vi "Main_Measurement.vi"(5 "error in":errorcluster) -> (19 "error out":errorcluster)   [LabVIEW 2011]
uses:
  Camera/lib/atmcd32d.llb/Shutter_type typedef.ctl
  Camera/lib/atmcd32d.llb/Shutter_mode typedef.ctl
  Camera/lib/atmcd32d.llb/Spool_method typedef.ctl
  Camera/lib/atmcd32d.llb/OutputAmplifier_type typedef.ctl
  Camera/lib/atmcd32d.llb/EMGainMode_mode typedef.ctl
  Camera/lib/atmcd32d.llb/Error Code Enum typedef.ctl
  Camera/lib/atmcd32d.llb/AcquisitionMode_mode typedef.ctl
  Camera/lib/atmcd32d.llb/ReadMode_mode typedef.ctl
  Camera/lib/atmcd32d.llb/TriggerMode_mode typedef.ctl
  Utilities/controls/ctlSeqFNs_PI_SysNr.ctl
  Variables/GlobalSetGetPixelOfRoi.vi
  Variables/ScanDirection.vi
  Variables/IlluminationPatterns.vi
  Variables/GlobalSetGetTriggerForPointMeasurement.vi
  Variables/GlobalDevice.vi
  Kinetics/vi/RampOrLin.vi
  Variables/MesaurementType.vi
  Variables/GlobalSetNumberOfDigits_PhysikalInstruments.vi
  Variables/GlobalSetNumberOfDigits_Scanners.vi
  Variables/ccdChipPixels.vi
  Variables/GlobalSetGetConfigureCamera.vi
  Variables/GlobalGetTimingsFromCamera.vi
  Variables/SavPath.vi
  Variables/GlobalSetConfigurationPhysikalInstruments.vi
  Variables/GlobalSetGetPositionParameters.vi
  <vilib>/DAQmx/create/channels.llb/DAQmx Create Channel (CO-Pulse Generation-Frequency).vi
  <vilib>/DAQmx/configure/timing.llb/DAQmx Timing (Implicit).vi
  <vilib>/DAQmx/configure/trigger.llb/DAQmx Start Trigger (Digital Edge).vi
  Variables/Pulsecounter.vi
  Variables/ModulationNiveaus.vi
  Variables/AOTF_NonLinearLinesOnOff.vi
  Variables/MesaurementTime.vi
  Program Files/National Instruments/LabVIEW 2011/resource/objmgr/daqmx.rc
panel:
  out "first":u32
  out "last":i32
  out "ypixels":i32
  out "xpixels":i32
  out "keepCleanTime":sgl
types:
  T1 = enum32{"Non Linear Illumniation", "Constant Illumination"}
  T2 = typedef "Shutter_type typedef.ctl" = enum16{"TTL Low", "TTL High"}
  T3 = typedef "Shutter_mode typedef.ctl" = enum16{"Auto", "Open", "Close"}
  T4 = typedef "Spool_method typedef.ctl" = enum16{"32-bit", "Depends", "16-bit", "Multiple Directory", "Spool to RAM disk", "16-bit FITS", "SIF", "16-buit TIFF", "Multiple Directory Compressed"}
  T5 = typedef "Error Code Enum typedef.ctl" = enum32{"N/A (0)", "DRV_ERROR_CODES", "DRV_SUCCESS", "DRV_VXDNOTINSTALLED", "DRV_ERROR_SCAN", "DRV_ERROR_CHECK_SUM", "DRV_ERROR_FILELOAD", "DRV_UNKNOWN_FUNC", "DRV_ERROR_VXD_INIT", "DRV_ERROR_ADDRESS", "DRV_ERROR_PAGELOCK", "DRV_ERROR_PAGEUNLOCK", "DRV_ERROR_BOARDTEST", "DRV_ERROR_ACK", "DRV_ERROR_UP_FIFO", "DRV_ERROR_PATTERN", "N/A (16)", "DRV_ACQUISITION_ERRORS", "DRV_ACQ_BUFFER", "DRV_ACQ_DOWNFIFO_FULL", "DRV_PROC_UNKONWN_INSTRUCTION", "DRV_ILLEGAL_OP_CODE", "DRV_KINETIC_TIME_NOT_MET", "DRV_ACCUM_TIME_NOT_MET", "DRV_NO_NEW_DATA", "N/A (25)", "DRV_SPOOLERROR", "N/A (27)", "N/A (28)", "N/A (29)", "N/A (30)", "N/A (31)", "N/A (32)", "DRV_TEMPERATURE_CODES", "DRV_TEMPERATURE_OFF", "DRV_TEMPERATURE_NOT_STABILIZED", "DRV_TEMPERATURE_STABILIZED", "DRV_TEMPERATURE_NOT_REACHED", "DRV_TEMPERATURE_OUT_RANGE", "DRV_TEMPERATURE_NOT_SUPPORTED", "DRV_TEMPERATURE_DRIFT", "N/A (41)", "N/A (42)", "N/A (43)", "N/A (44)", "N/A (45)", "N/A (46)", "N/A (47)", "N/A (48)", "DRV_GENERAL_ERRORS", "DRV_INVALID_AUX", "DRV_COF_NOTLOADED", "DRV_FPGAPROG", "DRV_FLEXERROR", "DRV_GPIBERROR", "N/A (55)", "N/A (56)", "N/A (57)", "N/A (58)", "N/A (59)", "N/A (60)", "N/A (61)", "N/A (62)", "N/A (63)", "DRV_DATATYPE", "DRV_DRIVER_ERRORS", "DRV_P1INVALID", "DRV_P2INVALID", "DRV_P3INVALID", "DRV_P4INVALID", "DRV_INIERROR", "DRV_COFERROR", "DRV_ACQUIRING", "DRV_IDLE", "DRV_TEMPCYCLE", "DRV_NOT_INITIALIZED", "DRV_P5INVALID", "DRV_P6INVALID", "DRV_INVALID_MODE", "DRV_INVALID_FILTER", "DRV_I2CERRORS", "DRV_I2CDEVNOTFOUND", "DRV_I2CTIMEOUT", "DRV_P7INVALID", "N/A (84)", "N/A (85)", "N/A (86)", "N/A (87)", "N/A (88)", "N/A (89)", "DRV_IOCERROR", "DRV_VRMVERSIONERROR"}
  T6 = typedef "OutputAmplifier_type typedef.ctl" = enum16{"Standard EMCCD gain register", "Conventional CCD register"}
  T7 = typedef "EMGainMode_mode typedef.ctl" = enum16{"8-bit", "12-bit", "Linear", "Real"}
  T8 = typedef "TriggerMode_mode typedef.ctl" = enum16{"Internal", "External", "N/A (2)", "N/A (3)", "N/A (4)", "N/A (5)", "External Start"}
  T9 = typedef "AcquisitionMode_mode typedef.ctl" = enum16{"Reserved (0)", "Single Scan", "Accumulate", "Kinetics", "Fast Kinetics", "Run Till Abort", "Reserved (6)", "Reserved (7)", "Reserved (8)", "Time Delayed Integration"}
  T10 = typedef "ReadMode_mode typedef.ctl" = enum16{"Full Vertical Binning", "Multi-Track", "Random-Track", "Single-Track", "Image"}
  T11 = typedef "ctlSeqFNs_PI_SysNr.ctl" = enum16{"Zero", "E517", "E710"}
  T12 = enum16{"open", "replace", "create", "open or create", "replace or create", "replace or create with confirmation"}
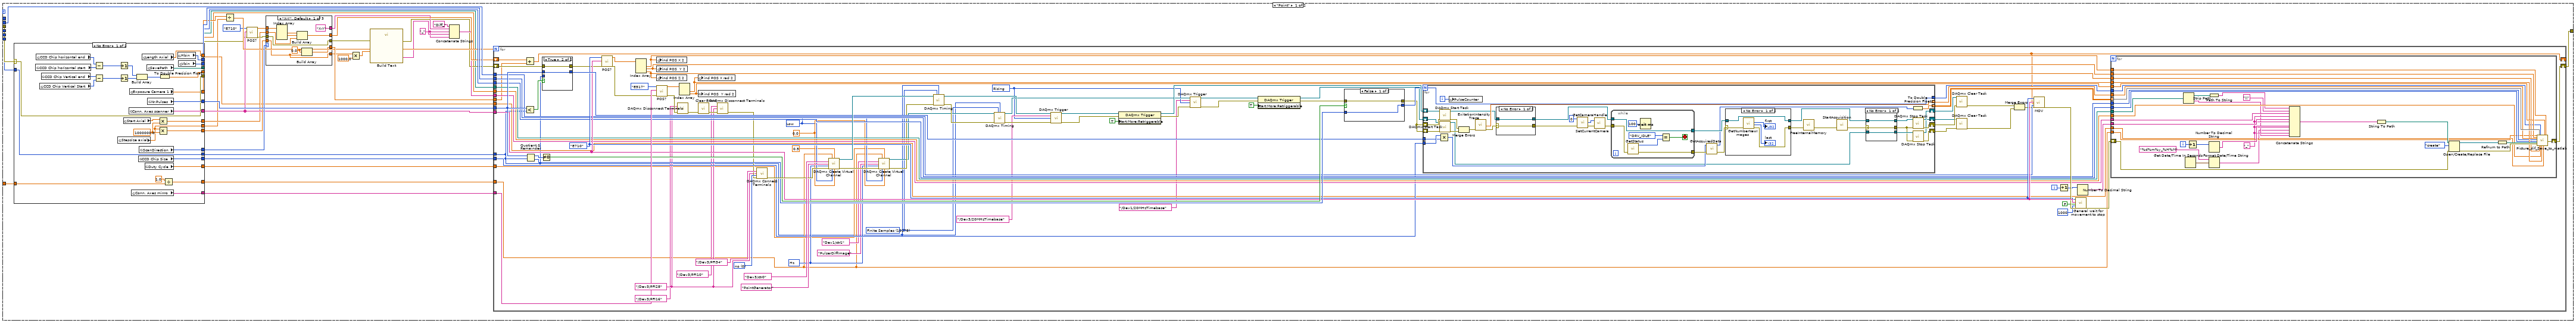
[diagram p2: hidden frame]
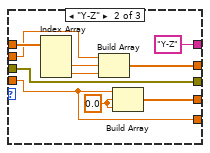
[diagram p3: hidden frame]
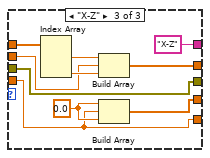
[diagram p4: hidden frame]
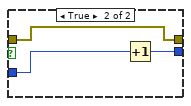
[diagram p6: hidden frame]
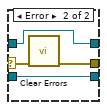
[diagram p7: hidden frame]
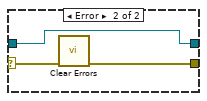
[diagram p8: hidden frame]
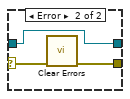
[diagram p9: hidden frame]
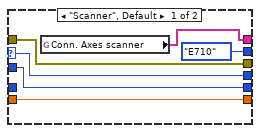
[diagram p11: hidden frame]
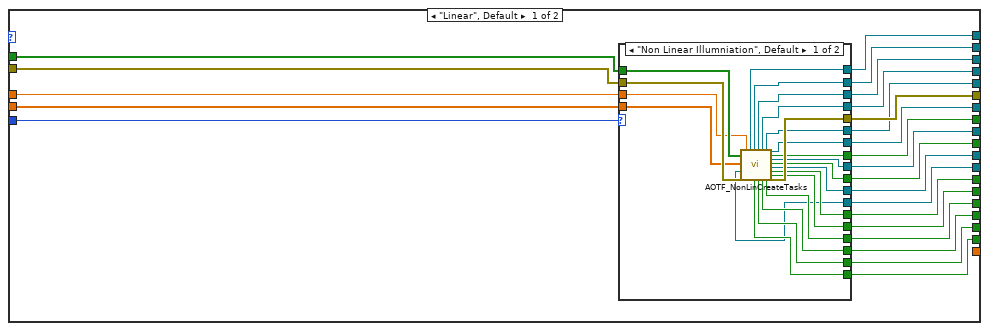
[diagram p14: hidden frame]
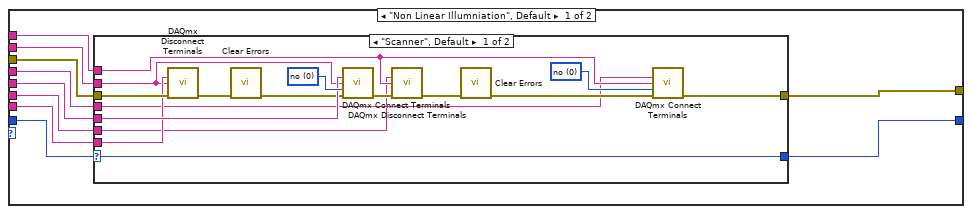
[diagram p17: hidden frame]
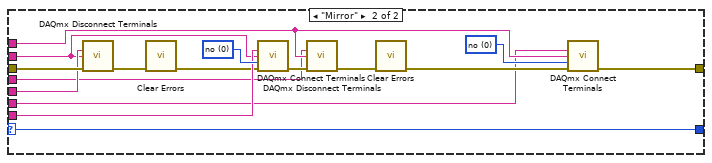
[diagram p18: hidden frame]
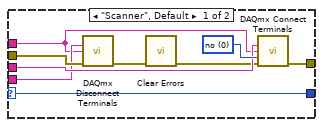
[diagram p19: hidden frame]
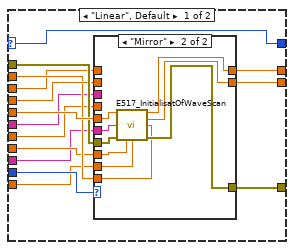
[diagram p20: hidden frame]
diagram:
  n1 = case shown="No Error" "error in" {
    selector: "error in" -> [w60 _]
    tunnel: [w71 _] -> w42
    tunnel: [w70 _] -> w41
    tunnel: [w69 _] -> w40
    tunnel: [w68 _] -> w39
    tunnel: [w67 _] -> w38
    tunnel: [w66 _] -> w37
    tunnel: [w65 _] -> w36
    tunnel: [0 ("camerahandler") _] -> w34
    tunnel: [w64 _] -> w33
    tunnel: [w63 _] -> w32
    tunnel: [w62 _] -> w23
    tunnel: [w61 _] -> w22
    tunnel: [w60 _] -> w30
    tunnel: [w58 _] -> w28
    tunnel: [w57 _] -> w26
    tunnel: [w56 _] -> w25
    tunnel: [w54 _] -> w15
    tunnel: [w52 _] -> w20
    tunnel: [w51 _] -> w19
    tunnel: [w49 _] -> w7
    tunnel: [w48 _] -> w6
    tunnel: [w47 _] -> w5
    tunnel: [w46 _] -> w4
    tunnel: [w45 _] -> w3
    tunnel: [w44 _] -> w2
    tunnel: [w43 _] -> w1
    frame No Error {
      n2 = global read "GlobalSetGetPixelOfRoi.vi" "Pixel SizeX"() -> (w68:dbl)
      n3 = global read "GlobalSetGetPixelOfRoi.vi" "Pixel SizeZ"() -> (w43:dbl)
      n4 = global read "GlobalSetGetPixelOfRoi.vi" "Pixel SizeY"() -> (w47:dbl)
      n5 = global read "GlobalSetGetPixelOfRoi.vi" "Pixel SizeZ"() -> (w46:dbl)
      n6 = global read "GlobalSetGetTriggerForPointMeasurement.vi" "Nr.Pulses"() -> (w53:i32)
      n7 = global read "GlobalSetGetConfigureCamera.vi" "Exposure"() -> (w71:sgl)
      n8 = global read "GlobalSetGetPixelOfRoi.vi" "X length"() -> (w67:dbl)
      n9 = global read "GlobalSetGetPixelOfRoi.vi" "Y length"() -> (w66:dbl)
      n10 = global read "MesaurementType.vi" "mesaurement type"() -> (w56:enum32{"Point", "Area"})
      n11 = global read "RampOrLin.vi" "Kinetice chooser"() -> (w52:enum32{"Linear", "Stepwise"})
      n12 = global read "ccdChipPixels.vi" "CCD Chip horizontal start"() -> (w64:i32)
      n13 = global read "ccdChipPixels.vi" "CCD Chip horizontal end"() -> (w62:i32)
      n14 = global read "GlobalSetNumberOfDigits_Scanners.vi" "NumberOfDigits Scanner"() -> (w58:i32)
      n15 = global read "GlobalDevice.vi" "Device Choser"() -> (w51:enum32{"Scanner", "Mirror"})
      n16 = global read "ScanDirection.vi" "ScanDirection"() -> (w48:enum32{"X-Y", "X-Z", "Y-Z", "Focus"})
      n17 = global read "GlobalSetNumberOfDigits_PhysikalInstruments.vi" "NumberOfDigits Mirror"() -> (w57:i32)
      n18 = global read "ccdChipPixels.vi" "CCD Chip Vertical Start"() -> (w63:i32)
      n19 = global read "ccdChipPixels.vi" "CCD Chip Vertical end"() -> (w61:i32)
      n20 = global read "GlobalSetGetPixelOfRoi.vi" "Stack length"() -> (w44:dbl)
      n21 = global read "GlobalSetGetPixelOfRoi.vi" "Stack length"() -> (w45:dbl)
      n22 = global read "GlobalSetGetTriggerForPointMeasurement.vi" "PulseSequenzelength"() -> (w50:i32)
      n23 = global read "IlluminationPatterns.vi" "Illumination Patterns"() -> (w49:T1)
      n24 = Less?(x=w53, y=w50) -> (x < y?=w55:bool)
      n25 = case shown="True" w55 {
        tunnel: [w72 w73] -> w54
        tunnel: w53 -> [_ w73]
        tunnel: w50 -> [w72 _]
        frame False {
        }
        frame True {
        }
      }
      n26 = global read "GlobalSetGetConfigureCamera.vi" "Hbin"() -> (w69:i32)
      n27 = global read "GlobalSetGetConfigureCamera.vi" "gain"() -> (w65:i32)
      n28 = global read "GlobalSetGetConfigureCamera.vi" "Vbin"() -> (w70:i32)
    }
    frame Error {
    }
  }
  n29 = case shown="No Error" w30 {
    selector: w30 -> [w131 _]
    tunnel: w42 -> [w165 _]
    tunnel: [w166 _] -> w12
    tunnel: w40 -> [w116 _]
    tunnel: w41 -> [w117 _]
    tunnel: w39 -> [w101 _]
    tunnel: w38 -> [w102 _]
    tunnel: w37 -> [w84 _]
    tunnel: [w136 _] -> w13
    tunnel: w36 -> [w164 _]
    tunnel: [w135 _] -> w35
    tunnel: w34 -> [w134 _]
    tunnel: w33 -> [w133 _]
    tunnel: w32 -> [w132 _]
    tunnel: [w122 _] -> w29
    tunnel: w28 -> [w122 _]
    tunnel: [w121 _] -> w27
    tunnel: w26 -> [w121 _]
    tunnel: w25 -> [w93 _]
    tunnel: [w93 _] -> w24
    tunnel: w15 -> [w92 _]
    tunnel: [w118 _] -> w14
    tunnel: w23 -> [w109 _]
    tunnel: w22 -> [w110 _]
    tunnel: w20 -> [w100 _]
    tunnel: w19 -> [w89 _]
    tunnel: [w90 _] -> w18
    tunnel: [w94 _] -> w17
    tunnel: [w91 _] -> w16
    tunnel: w7 -> [w86 _]
    tunnel: w6 -> [w74 _]
    tunnel: w5 -> [w83 _]
    tunnel: w4 -> [w80 _]
    tunnel: w3 -> [w79 _]
    tunnel: w2 -> [w76 _]
    tunnel: w1 -> [w75 _]
    frame No Error {
      w96 = 0 ("closingtime")
      n30 = Divide(x=w76, y=w75) -> (x/y=w77:dbl)
      n31 = Divide(x=w102, y=w101) -> (x/y=w82:dbl)
      n32 = Divide(x=w84, y=w83) -> (x/y=w81:dbl)
      n33 = Divide(x=w79, y=w80) -> (x/y=w78:dbl)
      n34 = call "GetCameraHandle.vi"("error in (no error)"=w131, "cameraIndex"=w134) -> ("error out"=w162:errorcluster, "cameraHandle"=w163:i32)  [unwired: 1 in, 1 out]
      n35 = call "SetCurrentCamera.vi"("error in (no error)"=w162, "cameraHandle"=w163) -> ("error out"=w161:errorcluster)  [unwired: 1 out]
      n36 = call "GetStatus.vi"("error in (no error)"=w161) -> ("error out"=w87:errorcluster, "status"=w159:T5)  [unwired: 2 in, 1 out]
      n37 = Not Equal?(x=Error_Code_Enum_typedef."DRV_IDLE" ("status"), y=w159) -> (x != y?=w158:bool)
      n38 = case shown="\"Constant Illumination\"" w86 {
        tunnel: w89 -> [_ w177]
        tunnel: w74 -> [_ w176]
        tunnel: [w168 w175] -> w88
        tunnel: w87 -> [w168 w174]
        tunnel: [w167 w173] -> w85
        tunnel: w82 -> [w167 w172]
        tunnel: w81 -> [_ w171]
        tunnel: w78 -> [_ w170]
        tunnel: w77 -> [_ w169]
        frame "Non Linear Illumniation", Default {
        }
        frame "Constant Illumination" {
          n39 = case shown="\"Scanner\", Default" w177 {
            tunnel: w176 -> [w183 _]
            tunnel: [w185 w195] -> w175
            tunnel: w174 -> [w184 w195]
            tunnel: [w182 w194] -> w173
            tunnel: w172 -> [w179 w194]
            tunnel: w171 -> [w180 _]
            tunnel: w170 -> [w181 _]
            tunnel: w169 -> [w178 _]
            frame "Scanner", Default {
              n40 = case shown="\"Focus\"" w183 {
                tunnel: [w187 w189 w190 w193] -> w185
                tunnel: w184 -> [w187 w189 w190 w193]
                tunnel: [w186 w188 w191 w192] -> w182
                tunnel: w181 -> [_ _ _ _]
                tunnel: w180 -> [_ _ _ w192]
                tunnel: w179 -> [w186 w188 _ _]
                tunnel: w178 -> [_ _ w191 _]
                frame "X-Y", Default {
                }
                frame "X-Z" {
                }
                frame "Focus" {
                }
                frame "Y-Z" {
                }
              }
            }
            frame "Mirror" {
            }
          }
        }
      }
      n41 = case shown="False" w158 {
        tunnel: w88 -> [w259 w261]
        tunnel: [w259 w260] -> w155
        frame False {
        }
        frame True {
          n42 = call "AbortAcquisition.vi"("error in (no error)"=w261) -> ("error out"=w260:errorcluster)  [unwired: 1 in, 1 out]
        }
      }
      n43 = call "GetDetector.vi"("error in (no error)"=w155) -> ("error out"=w156:errorcluster, "ypixels"=→"ypixels":i32, "xpixels"=→"xpixels":i32)  [unwired: 3 in, 1 out]
      n44 = call "FreeInternalMemory.vi"("error in (no error)"=w156) -> ("error out"=w120:errorcluster)  [unwired: 1 in, 1 out]
      n45 = case shown="\"Linear\"" w100 {
        selector: w100 -> [w233 _]
        tunnel: [w238 w243] -> w124
        tunnel: w120 -> [w237 w242]
        tunnel: w89 -> [w234 w241]
        tunnel: [w234 w240] -> w90
        tunnel: [w233 _] -> w99
        frame "Stepwise", Default {
          n46 = call "SetAcquisitionMode.vi"("error in (no error)"=w237, "mode"=AcquisitionMode_mode_typedef."Single Scan") -> ("error out"=w236:errorcluster)  [unwired: 1 out]
          n47 = call "SetReadMode.vi"("error in (no error)"=w236, "mode"=ReadMode_mode_typedef."Image") -> ("error out"=w238:errorcluster)  [unwired: 1 out]
        }
        frame "Linear" {
          n48 = case shown="\"Scanner\", Default" w241 {
            selector: w241 -> [w244 w250]
            tunnel: [w248 w254] -> w243
            tunnel: w242 -> [w247 w253]
            tunnel: [w244 w250] -> w240
            frame "Scanner", Default {
              n49 = call "SetAcquisitionMode.vi"("error in (no error)"=w247, "mode"=AcquisitionMode_mode_typedef."Kinetics") -> ("error out"=w246:errorcluster)  [unwired: 1 out]
              n50 = call "SetReadMode.vi"("error in (no error)"=w246, "mode"=ReadMode_mode_typedef."Image") -> ("error out"=w248:errorcluster)  [unwired: 1 out]
            }
            frame "Mirror" {
              n51 = call "SetAcquisitionMode.vi"("error in (no error)"=w253, "mode"=AcquisitionMode_mode_typedef."Kinetics") -> ("error out"=w252:errorcluster)  [unwired: 1 out]
              n52 = call "SetReadMode.vi"("error in (no error)"=w252, "mode"=ReadMode_mode_typedef."Image") -> ("error out"=w254:errorcluster)  [unwired: 1 out]
            }
          }
        }
      }
      n53 = call "GetStatus.vi"("error in (no error)"=w124) -> ("error out"=w125:errorcluster, "status"=w127:T5)  [unwired: 2 in, 1 out]
      n54 = Not Equal?(x=Error_Code_Enum_typedef."DRV_IDLE" ("status"), y=w127) -> (x != y?=w126:bool)
      n55 = case shown="False" w126 {
        tunnel: w125 -> [w256 w258]
        tunnel: [w256 w257] -> w123
        frame False {
        }
        frame True {
          n56 = call "AbortAcquisition.vi"("error in (no error)"=w258) -> ("error out"=w257:errorcluster)  [unwired: 1 in, 1 out]
        }
      }
      n57 = call "SetImage.vi"("hbin"=w116, "vbin"=w117, "hstart"=w133, "hend"=w109, "vstart"=w132, "vend"=w110, "error in (no error)"=w123) -> ("error out"=w111:errorcluster)  [unwired: 19 in, 1 out]
      n58 = Boolean To (0,1)(Boolean=FALSE) -> (0, 1=w107:i16)
      n59 = call "SetIsolatedCropMode.vi"("hbin"=w116, "vbin"=w117, "error in (no error)"=w111, "cropWidth"=w109, "cropHeight"=w110, "active"=w107) -> ("error out"=w104:errorcluster)  [unwired: 1 out]
      n60 = call <vilib>:"Clear Errors.vi"("error in (no error)"=w104) -> ("error out"=w103:errorcluster)  [unwired: 6 in]
      n61 = call "SetSpool.vi"("active"=FALSE, "method"=Spool_method_typedef."32-bit", "name"="test", "framebuffersize (10)"=10, "error in (no error)"=w103) -> ("error out"=w98:errorcluster)  [unwired: 9 in, 1 out]
      n62 = case shown="\"Linear\", Default" w99 {
        tunnel: [w228 w231] -> w154
        tunnel: w98 -> [w225 w230]
        frame "Linear", Default {
          n63 = call "SetFastExtTrigger.vi"("error in (no error)"=w225, "mode"=TRUE) -> ("error out"=w226:errorcluster)  [unwired: 1 out]
          n64 = call "SetTriggerMode.vi"("error in (no error)"=w226, "mode"=TriggerMode_mode_typedef."External") -> ("error out"=w228:errorcluster)  [unwired: 1 out]
        }
        frame "Stepwise" {
          n65 = call "SetTriggerMode.vi"("error in (no error)"=w230, "mode"=TriggerMode_mode_typedef."Internal") -> ("error out"=w231:errorcluster)  [unwired: 1 out]
        }
      }
      n66 = call "SetFrameTransferMode.vi"("error in (no error)"=w154, "mode"=enum16{"OFF", "ON"}."ON") -> ("error out"=w137:errorcluster)  [unwired: 1 out]
      n67 = call "SetEMGainMode.vi"("error in (no error)"=w137, "mode"=EMGainMode_mode_typedef."Linear") -> ("error out"=w142:errorcluster)  [unwired: 1 out]
      n68 = call "SetEMCCDGain.vi"("error in (no error)"=w142, "gain"=w164) -> ("error out"=w141:errorcluster)  [unwired: 1 out]
      n69 = call "SetExposureTime.vi"("error in (no error)"=w141, "time"=w165) -> ("error out"=w140:errorcluster)  [unwired: 1 out]
      n70 = call "SetOutputAmplifier.vi"("error in (no error)"=w140, "type"=OutputAmplifier_type_typedef."Standard EMCCD gain register") -> ("error out"=w139:errorcluster)  [unwired: 1 out]
      n71 = call "SetADChannel.vi"("error in (no error)"=w139, "channel"=0) -> ("error out"=w152:errorcluster)  [unwired: 1 out]
      n72 = call "GetNumberVSSpeeds.vi"("error in (no error)"=w152) -> ("error out"=w151:errorcluster, "number"=w150:i32)  [unwired: 2 in, 1 out]
      n73 = Subtract(x=w150, y=1) -> (x-y=w148:i32)
      n74 = call "SetVSSpeed.vi"("error in (no error)"=w151, "index"=w148) -> ("error out"=w147:errorcluster)  [unwired: 1 out]
      n75 = case shown="\"Area\"" w93 {
        selector: w93 -> [w197 w204]
        tunnel: w147 -> [w200 w209]
        tunnel: [w199 w208] -> w146
        tunnel: w99 -> [w198 w207]
        tunnel: [w198 w206] -> w94
        tunnel: w92 -> [w196 w203]
        tunnel: [w197 w205] -> _
        tunnel: [w196 w203] -> w91
        tunnel: w86 -> [_ w202]
        tunnel: w85 -> [_ w201]
        frame "Point", Default {
          n76 = call "SetNumberKinetics.vi"("error in (no error)"=w200, "number"=w196) -> ("error out"=w199:errorcluster)  [unwired: 1 out]
        }
        frame "Area" {
          n77 = case shown="\"Linear\", Default" w207 {
            selector: w207 -> [w213 w223]
            tunnel: w209 -> [w215 w224]
            tunnel: [w214 w224] -> w208
            tunnel: [w213 w223] -> w206
            tunnel: [w212 w222] -> w205
            tunnel: w204 -> [w212 w222]
            tunnel: w202 -> [w211 _]
            tunnel: w201 -> [w210 _]
            frame "Linear", Default {
              n78 = case shown="\"Constant Illumination\"" w211 {
                tunnel: w215 -> [w218 w221]
                tunnel: [w217 w220] -> w214
                tunnel: w210 -> [w216 w219]
                frame "Non Linear Illumniation", Default {
                  n79 = call "SetNumberKinetics.vi"("error in (no error)"=w218, "number"=w216) -> ("error out"=w217:errorcluster)  [unwired: 1 out]
                }
                frame "Constant Illumination" {
                  n80 = call "SetNumberKinetics.vi"("error in (no error)"=w221, "number"=w219) -> ("error out"=w220:errorcluster)  [unwired: 1 out]
                }
              }
            }
            frame "Stepwise" {
            }
          }
        }
      }
      n81 = call "SetShutter.vi"("type"=Shutter_type_typedef."TTL High", "mode"=Shutter_mode_typedef."Open", "closingtime"=w96, "openingtime"=w96, "error in (no error)"=w146) -> ("error out"=w145:errorcluster)  [unwired: 9 in, 1 out]
      n82 = call "GetAcquisitionTimings.vi"("error in (no error)"=w145) -> ("exposure"=w118:sgl, "accumulate"=w135:sgl, "kinetic"=w136:sgl, "error out"=w144:errorcluster)  [unwired: 10 in, 1 out]
      n83 = call "GetKeepCleanTime.vi"("error in (no error)"=w144) -> ("error out"=w130:errorcluster, "keepCleanTime"=→"keepCleanTime":sgl)  [unwired: 4 in, 1 out]
      n84 = call "FreeInternalMemory.vi"("error in (no error)"=w130) -> ("error out"=w129:errorcluster)  [unwired: 1 in, 1 out]
      n85 = call "StartAcquisition.vi"("error in (no error)"=w129) -> ("error out"=w166:errorcluster)  [unwired: 1 in, 1 out]
    }
    frame Error {
    }
  }
  n86 = global write "GlobalGetTimingsFromCamera.vi" "Exposure Camera 1"(w14) -> ()
  n87 = global write "GlobalGetTimingsFromCamera.vi" "Accumulation Camera 1"(w35) -> ()
  n88 = global write "GlobalGetTimingsFromCamera.vi" "Kinetics Camera 1"(w13) -> ()
  n89 = global read "IlluminationPatterns.vi" "Illumination Patterns"() -> (w9:T1)
  n90 = case shown="\"Constant Illumination\"" w9 {
    tunnel: [w262 w264] -> w21
    tunnel: w12 -> [w262 w263]
    frame "Constant Illumination" {
    }
    frame "Non Linear Illumniation" {
      n91 = Concatenate Strings("daughter disable" ("string"), "\r") -> (w267:string)
      n92 = call "CTI_AOTF.vi"("error in"=w263, "String"=w267, "VISA resource name 2"=refnum<visa-resource-name> "USB0::0x16C7::0x0001::NI-VISA-20001::RAW") -> ("error out"=w264:errorcluster)  [unwired: 7 in, 1 out]
    }
  }
  n93 = case shown="\"Area\", Default" w24 {
    tunnel: w21 -> [w303 w593]
    tunnel: w29 -> [w297 w582]
    tunnel: w27 -> [_ w581]
    tunnel: [w304 w575] -> w11
    tunnel: w13 -> [w301 w576]
    tunnel: w18 -> [_ w579]
    tunnel: w17 -> [_ w578]
    tunnel: w16 -> [w300 _]
    frame "Point" {
      w278 = "_" ("string")
      n94 = case shown="No Error" w303 {
        selector: w303 -> [w565 w572]
        tunnel: [w571 _] -> w269
        tunnel: [w570 _] -> w307
        tunnel: [w569 _] -> w306
        tunnel: [w568 _] -> w305
        tunnel: [w563 _] -> w298
        tunnel: [w567 _] -> w290
        tunnel: [w566 _] -> w302
        tunnel: [w565 w572] -> w288
        tunnel: w301 -> [w562 _]
        tunnel: w300 -> [w561 _]
        tunnel: [w561 _] -> w299
        tunnel: [w560 _] -> w294
        tunnel: [w559 _] -> w296
        tunnel: [w544 _] -> w293
        tunnel: [w545 _] -> w286
        tunnel: [w547 _] -> w277
        tunnel: [w549 _] -> w276
        tunnel: [w548 _] -> w275
        tunnel: [w542 _] -> w274
        tunnel: [w541 _] -> w270
        frame No Error {
          w543 = 1000000.0 ("y")
          n95 = global read "ccdChipPixels.vi" "CCD Chip horizontal start"() -> (w557:i32)
          n96 = global read "ccdChipPixels.vi" "CCD Chip horizontal end"() -> (w558:i32)
          n97 = global read "ccdChipPixels.vi" "CCD Chip Vertical Start"() -> (w555:i32)
          n98 = global read "ccdChipPixels.vi" "CCD Chip Vertical end"() -> (w556:i32)
          n99 = Subtract(x=w558, y=w557) -> (x-y=w552:i32)
          n100 = Subtract(x=w556, y=w555) -> (x-y=w551:i32)
          n101 = global read "GlobalSetGetPixelOfRoi.vi" "Stepsize axial"() -> (w542:dbl)
          n102 = Increment(x=w552) -> (x+1=w554:i32)
          n103 = Increment(x=w551) -> (x+1=w553:i32)
          n104 = global read "GlobalSetGetPixelOfRoi.vi" "Start Axial"() -> (w546:dbl)
          n105 = global read "GlobalSetConfigurationPhysikalInstruments.vi" "Conn. Axes scanner"() -> (w567:string[])
          n106 = global read "GlobalGetTimingsFromCamera.vi" "Exposure Camera 1"() -> (w541:dbl)
          n107 = global read "GlobalSetConfigurationPhysikalInstruments.vi" "Conn. Axes mirrro"() -> (w570:string[])
          n108 = Build Array(w554, w553) -> (w550:i32[])
          n109 = global read "ccdChipPixels.vi" "CCD Chip Size"() -> (w548:i32)
          n110 = global read "ScanDirection.vi" "ScanDirection"() -> (w560:enum32{"X-Y", "X-Z", "Y-Z", "Focus"})
          n111 = global read "GlobalSetGetPixelOfRoi.vi" "Length Axial"() -> (w559:dbl)
          n112 = global read "GlobalSetGetTriggerForPointMeasurement.vi" "Duty Cycle"() -> (w571:dbl)
          n113 = global read "SavPath.vi" "SavePath"() -> (w547:path)
          n114 = global read "GlobalSetGetTriggerForPointMeasurement.vi" "Nr.Pulses"() -> (w566:i32)
          n115 = Multiply(x=w546, y=w543) -> (x*y=w545:dbl)
          n116 = Multiply(x=w542, y=w543) -> (x*y=w544:dbl)
          n117 = To Double Precision Float(number=w550) -> (double precision float=w549:dbl[])
          n118 = Divide(x=sgl 1.0, y=w562) -> (x/y=w563:sgl)
          n119 = global read "GlobalSetGetConfigureCamera.vi" "Hbin"() -> (w569:i32)
          n120 = global read "GlobalSetGetConfigureCamera.vi" "Vbin"() -> (w568:i32)
        }
        frame Error {
        }
      }
      n121 = Divide(x=w296, y=w274) -> (x/y=w292:dbl)
      n122 = call "POS?.vi"("System no."=ctlSeqFNs_PI_SysNr."E710" ("DeviceNr."), "Axes to query"=w290, "error in"=w288) -> ("Position"=w287:dbl[], "error out"=w289:errorcluster)  [unwired: 15 in]
      n123 = case shown="\"X-Y\", Default" w294 {
        tunnel: w289 -> [w316 w326 w336]
        tunnel: [w316 w326 w336] -> w280
        tunnel: [w317 w327 w337] -> w295
        tunnel: w293 -> [w308 w318 w328]
        tunnel: w287 -> [w313 w322 w334]
        tunnel: w286 -> [w311 w320 w331]
        tunnel: [w310 w323 w330] -> w285
        tunnel: ["X-Y" "Y-Z" "X-Z"] -> w284
        tunnel: [w308 w318 w328] -> w272
        frame "X-Y", Default {
          w315 = 0.0 ("element")
          n124 = Index Array(array=w313) -> (element #1=w314:dbl, element #2=w312:dbl)  [unwired: 3 in, 1 out]
          n125 = Build Array(w314, w312, w311) -> (w310:dbl[])
          n126 = Build Array(w315, w315, w308) -> (w317:dbl[])
        }
        frame "Y-Z" {
          w325 = 0.0 ("element")
          n127 = Index Array(array=w322) -> (element #2=w321:dbl, element #3=w324:dbl)  [unwired: 3 in, 1 out]
          n128 = Build Array(w320, w321, w324) -> (w323:dbl[])
          n129 = Build Array(w318, w325, w325) -> (w327:dbl[])
        }
        frame "X-Z" {
          w335 = 0.0 ("element")
          n130 = Index Array(array=w334) -> (element #1=w333:dbl, element #3=w332:dbl)  [unwired: 3 in, 1 out]
          n131 = Build Array(w333, w331, w332) -> (w330:dbl[])
          n132 = Build Array(w335, w328, w335) -> (w337:dbl[])
        }
      }
      n133 = Multiply(x=w272, y=1000.0) -> (x*y=w273:dbl)
      n134 = call "Build Text"("step"=w273, "error in (no error)"=w280) -> ("Result"=w281:string, "error out"=w279:errorcluster)  [unwired: 12 in]
      n135 = Concatenate Strings("Diff_" ("string"), w284, w278, w281, w278) -> (w282:string)
      n136 = for {
        N: w292 -> [_]
        tunnel: w307 -> [w422]
        tunnel: w306 -> [w381]
        tunnel: w305 -> [w382]
        tunnel: w269 -> [w347]
        tunnel: w302 -> [w401]
        tunnel: w299 -> [w345]
        tunnel: w298 -> [w346]
        tunnel: w290 -> [w399]
        tunnel: w297 -> [w394]
        shift-right: [w415] -> w304
        shift-left: w279 -> [w389]
        shift-right: [w390] -> _
        shift-left: w285 -> [w392]
        tunnel: w295 -> [w378]
        tunnel: w282 -> [w384]
        tunnel: w276 -> [w380]
        tunnel: w275 -> [w379]
        tunnel: w277 -> [w385]
        tunnel: w270 -> [w376]
        i -> [w387]
        w354 = 0.0 ("initial delay")
        w395 = ctlSeqFNs_PI_SysNr."E710" ("DeviceNr.")
        w355 = 10178 items=["Finite Samples"=10178, "Continuous Samples"=10123, "Hardware Timed Single Point"=12522] ("Mode")
        w352 = 10373 items=["Hz"=10373] ("units")
        w356 = 10280 items=["Rising"=10280, "Falling"=10171] ("Trigger Edge")
        w353 = 10214 items=["High"=10192, "Low"=10214] ("Idle State")
        w431 = 0 items=["no", "yes"] ("invert polarity")
        w371 = tag "/Dev3/PFI28" ("destination terminal")
        n137 = Add(x=w392, y=w378) -> (x+y=w390:dbl[])
        n138 = Less?(x=w401, y=w345) -> (x < y?=w400:bool)
        n139 = Quotient & Remainder(x=w401, y=w345) -> (x-y*floor(x/y)=w406:i32, floor(x/y)=w404:i32)
        n140 = Not Equal To 0?(x=w406) -> (x != 0?=w405:bool)
        n141 = case shown="True" w400 {
          tunnel: w345 -> [w433 _]
          tunnel: [w433 w435] -> w402
          tunnel: w401 -> [_ w435]
          tunnel: [w432 w434] -> w388
          tunnel: w389 -> [w432 w434]
          frame False {
          }
          frame True {
          }
        }
        n142 = call "POS?.vi"("System no."=w395, "Axes to query"=w399, "error in"=w388) -> ("Position"=w393:dbl[], "error out"=w421:errorcluster)  [unwired: 15 in]
        n143 = Index Array(array=w393) -> (element #1=w410:dbl, element #2=w412:dbl, element #3=w411:dbl)  [unwired: 3 in]
        n144 = global write "GlobalSetGetPositionParameters.vi" "ind POS X 2"(w410) -> ()
        n145 = global write "GlobalSetGetPositionParameters.vi" "ind POS  Y 2"(w412) -> ()
        n146 = global write "GlobalSetGetPositionParameters.vi" "ind POS Z 2"(w411) -> ()
        n147 = call "POS?.vi"("System no."=ctlSeqFNs_PI_SysNr."E517" ("DeviceNr."), "Axes to query"=w422, "error in"=w421) -> ("Position"=w419:dbl[], "error out"=w374:errorcluster)  [unwired: 15 in]
        n148 = call <vilib>:"DAQmx Disconnect Terminals.vi"("source terminal"=tag "/Dev3/PFI16", "destination terminal"=w371, "error in"=w374) -> ("error out"=w375:errorcluster)  [unwired: 12 in]
        n149 = Index Array(array=w419) -> (element #1=w408:dbl, element #2=w409:dbl)  [unwired: 2 in]
        n150 = global write "GlobalSetGetPositionParameters.vi" "ind POS X rad 2"(w408) -> ()
        n151 = global write "GlobalSetGetPositionParameters.vi" "ind POS  Y rad 2"(w409) -> ()
        n152 = call <vilib>:"Clear Errors.vi"("error in (no error)"=w375) -> ("error out"=w373:errorcluster)  [unwired: 6 in]
        n153 = call <vilib>:"DAQmx Disconnect Terminals.vi"("source terminal"=tag "/Dev3/PFI10", "destination terminal"=w371, "error in"=w373) -> ("error out"=w372:errorcluster)  [unwired: 12 in]
        n154 = call <vilib>:"DAQmx Connect Terminals.vi"("source terminal"=tag "/Dev3/PFI34", "destination terminal"=w371, "invert polarity"=w431, "error in"=w372) -> ("error out"=w423:errorcluster)  [unwired: 11 in]
        n155 = call-poly <vilib>:"DAQmx Create Virtual Channel.vi"("frequency"=w346, "duty cycle"=0.5, "counter"=tag "Dev3/ctr0", "name to assign"="PointGenerator", "units"=w352, "error in"=w423, "idle state"=w353, "initial delay"=w354) -> ("task out"=w424:refnum<k21>, "error out"=w368:errorcluster)  [unwired: 6 in]
        n156 = call-poly <vilib>:"DAQmx Create Virtual Channel.vi"("frequency"=w346, "duty cycle"=w347, "counter"=tag "Dev1/ctr1", "name to assign"="PulserDiffImage", "units"=w352, "error in"=w368, "idle state"=w353, "initial delay"=w354) -> ("task out"=w364:refnum<k21>, "error out"=w367:errorcluster)  [unwired: 6 in]
        n157 = call-poly <vilib>:"DAQmx Timing.vi"("task/channels in"=w424, "sample mode"=w355, "samples per channel"=w345, "error in"=w367) -> ("task out"=w425:refnum<k21>, "error out"=w366:errorcluster)  [unwired: 10 in]
        n158 = call-poly <vilib>:"DAQmx Timing.vi"("task/channels in"=w364, "sample mode"=w355, "samples per channel"=w345, "error in"=w366) -> ("task out"=w358:refnum<k21>, "error out"=w365:errorcluster)  [unwired: 10 in]
        n159 = call-poly <vilib>:"DAQmx Trigger.vi"("task/channels in"=w425, "source"=tag "/Dev3/20MHzTimebase", "edge"=w356, "error in"=w365) -> ("task out"=w426:refnum<k21>, "error out"=w427:errorcluster)  [unwired: 10 in]
        n160 = property class="DAQmx Trigger"(reference=w426, error in=w427, "Start:More:Retriggerable"=TRUE) -> (reference out=w418:refnum<k21>, error out=w361:errorcluster)
        n161 = call-poly <vilib>:"DAQmx Trigger.vi"("task/channels in"=w358, "source"=tag "/Dev1/20MHzTimebase", "edge"=w356, "error in"=w361) -> ("task out"=w359:refnum<k21>, "error out"=w362:errorcluster)  [unwired: 10 in]
        n162 = property class="DAQmx Trigger"(reference=w359, error in=w362, "Start:More:Retriggerable"=TRUE) -> (reference out=w340:refnum<k21>, error out=w360:errorcluster)
        n163 = case shown="False" w405 {
          tunnel: w404 -> [w437 w440]
          tunnel: [w437 w439] -> w403
          tunnel: [w436 w438] -> w344
          tunnel: w360 -> [w436 w438]
          frame False {
          }
          frame True {
            n164 = Increment(x=w440) -> (x+1=w439:i32)
          }
        }
        n165 = for {
          N: w403 -> [w489]
          shift-right: [w479] -> w417
          shift-left: w344 -> [w513]
          shift-right: [w497] -> w416
          shift-left: w418 -> [w487]
          tunnel: w379 -> [w504]
          tunnel: [w506] -> w414 mode=indexing
          tunnel: [w491] -> w413 mode=indexing
          tunnel: w402 -> [w502]
          tunnel: [w489] -> w377
          shift-right: [w478] -> w342
          shift-left: w344 -> [w486]
          shift-right: [w477] -> w341
          shift-left: w340 -> [w476]
          i -> [w488]
          n166 = Multiply(x=w504, y=w502) -> (x*y=w498:i32)
          n167 = call <vilib>:"DAQmx Start Task.vi"("task/channels in"=w487, "error in"=w513) -> ("task out"=w496:refnum<k21>, "error out"=w484:errorcluster)  [unwired: 12 in]
          n168 = call <vilib>:"DAQmx Start Task.vi"("task/channels in"=w476, "error in"=w486) -> ("task out"=w482:refnum<k21>, "error out"=w485:errorcluster)  [unwired: 12 in]
          n169 = global write "Pulsecounter.vi" "PulseCounter"(w488) -> ()
          n170 = Merge Errors(w484, w485) -> (w483:errorcluster)
          n171 = call "ExitationIntensityTrace.vi"("error in 2"=w483) -> ("data"=w506:dbl, "error out"=w505:errorcluster)  [unwired: 17 in]
          n172 = case shown="No Error" w505 {
            selector: w505 -> [w537 w540]
            tunnel: [w537 w539] -> w501
            tunnel: w496 -> [w536 w538]
            tunnel: [w536 w538] -> w495
            frame No Error {
            }
            frame Error {
              n173 = call <vilib>:"Clear Errors.vi"("error in (no error)"=w540) -> ("error out"=w539:errorcluster)  [unwired: 6 in]
            }
          }
          n174 = call "GetCameraHandle.vi"("error in (no error)"=w501, "cameraIndex"=0) -> ("error out"=w511:errorcluster, "cameraHandle"=w512:i32)  [unwired: 1 in, 1 out]
          n175 = call "SetCurrentCamera.vi"("error in (no error)"=w511, "cameraHandle"=w512) -> ("error out"=w500:errorcluster)  [unwired: 1 out]
          n176 = while {
            tunnel: [w518] -> w499
            tunnel: w500 -> [w517]
            tunnel: w495 -> [w514]
            tunnel: [w514] -> w494
            stop <- w516 stop-if-true
            n177 = call "GetStatus.vi"("error in (no error)"=w517) -> ("error out"=w518:errorcluster, "status"=w519:T5)  [unwired: 2 in, 1 out]
            n178 = Wait (ms)(milliseconds to wait=u32 100) -> ()  [unwired: 1 out]
            n179 = Equal?(x=Error_Code_Enum_typedef."DRV_IDLE" ("status"), y=w519) -> (x = y?=w516:bool)
          }
          n180 = call "GetAcquiredData.vi"("error in (no error)"=w499, "size"=w498) -> ("error out"=w503:errorcluster, "array"=w490:i32[])  [unwired: 1 in, 1 out]
          n181 = case shown="No Error" w503 {
            selector: w503 -> [w531 w535]
            tunnel: [w530 w534] -> w508
            tunnel: w494 -> [w532 w533]
            tunnel: [w532 w533] -> w493
            frame No Error {
              n182 = call "GetNumberNewImages.vi"("error in (no error)"=w531) -> ("error out"=w530:errorcluster, "last"=→"last":i32, "first"=→"first":u32)  [unwired: 3 in, 1 out]
            }
            frame Error {
              n183 = call <vilib>:"Clear Errors.vi"("error in (no error)"=w535) -> ("error out"=w534:errorcluster)  [unwired: 6 in]
            }
          }
          n184 = call "FreeInternalMemory.vi"("error in (no error)"=w508) -> ("error out"=w509:errorcluster)  [unwired: 1 in, 1 out]
          n185 = call "StartAcquisition.vi"("error in (no error)"=w509) -> ("error out"=w507:errorcluster)  [unwired: 1 in, 1 out]
          n186 = case shown="No Error" w507 {
            selector: w507 -> [w523 w527]
            tunnel: [w523 w526] -> w480
            tunnel: w493 -> [w522 w525]
            tunnel: [w522 w525] -> w492
            tunnel: w482 -> [w521 w524]
            tunnel: [w521 w524] -> w481
            frame No Error {
            }
            frame Error {
              n187 = call <vilib>:"Clear Errors.vi"("error in (no error)"=w527) -> ("error out"=w526:errorcluster)  [unwired: 6 in]
            }
          }
          n188 = To Double Precision Float(number=w490) -> (double precision float=w491:dbl[])
          n189 = call <vilib>:"DAQmx Stop Task.vi"("task/channels in"=w492, "error in"=w480) -> ("task out"=w497:refnum<k21>, "error out"=w479:errorcluster)  [unwired: 12 in]
          n190 = call <vilib>:"DAQmx Stop Task.vi"("task/channels in"=w481, "error in"=w480) -> ("task out"=w477:refnum<k21>, "error out"=w478:errorcluster)  [unwired: 12 in]
        }
        n191 = call <vilib>:"DAQmx Clear Task.vi"("task in"=w416, "error in"=w417) -> ("error out"=w343:errorcluster)  [unwired: 13 in]
        n192 = call <vilib>:"DAQmx Clear Task.vi"("task in"=w341, "error in"=w342) -> ("error out"=w339:errorcluster)  [unwired: 13 in]
        n193 = Merge Errors(w343, w339) -> (w338:errorcluster)
        n194 = call "MOV.vi"("System no."=w395, "Axes to move"=w399, "Position values"=w390, "No.of digits"=w394, "error in"=w338) -> ("error out"=w398:errorcluster)  [unwired: 14 in]
        n195 = Increment(x=w387) -> (x+1=w386:i32)
        n196 = call "General wait for movement to stop.vi"("System no."=w395, "Axes to wait for"=w399, "All axes?"=FALSE, "Additional wait time, ms"=u32 1000, "error in"=w398) -> ("error out"=w391:errorcluster)  [unwired: 13 in, 1 out]
        n197 = Number To Decimal String(number=w386) -> (decimal integer string=w383:string)  [unwired: 1 in]
        n198 = for {
          shift-right: [w466] -> w415
          shift-left: w391 -> [w462]
          tunnel: w413 -> [w473] mode=indexing
          tunnel: w414 -> [w472]
          tunnel: w409 -> [w464]
          tunnel: w408 -> [w463]
          tunnel: w384 -> [w459]
          tunnel: w383 -> [w458]
          tunnel: w382 -> [w454]
          tunnel: w381 -> [w453]
          tunnel: w380 -> [w451]
          tunnel: w410 -> [w470]
          tunnel: w412 -> [w471]
          tunnel: w411 -> [w452]
          tunnel: w346 -> [w450]
          tunnel: w385 -> [w456]
          tunnel: w377 -> [w442]
          tunnel: w376 -> [w441]
          i -> [w475]
          w449 = "_" ("string")
          n199 = Strip Path(path=w456) -> (stripped path=w455:path, name=w448:string)
          n200 = Get Date/Time In Seconds() -> (seconds since 1Jan1904=w446:timestamp)
          n201 = Increment(x=w475) -> (x+1=w474:i32)
          n202 = Path To String(path=w455) -> (string=w444:string)
          n203 = Number To Decimal String(number=w474) -> (decimal integer string=w457:string)  [unwired: 1 in]
          n204 = Format Date/Time String(time format string (%c)="%d%m%y_%H%M", seconds (now)=w446) -> (date/time string=w445:string)  [unwired: 1 in]
          n205 = Concatenate Strings(w444, "\\" ("string"), w459, w449, w458, w449, w457, w449, w445, w449, w448) -> (w461:string)
          n206 = String To Path(string=w461) -> (path=w460:path)
          n207 = Open/Create/Replace File(file path (use dialog)=w460, error in=w462, operation (0:open)=T12."create") -> (refnum out=w468:refnum<file>, error out=w467:errorcluster)  [unwired: 4 out]
          n208 = Refnum to Path(1:w468) -> (0:w465:path)
          n209 = call "Picture_dif_Save_to_matlab.vi"("Frequency"=w450, "Pos_Y_Sca"=w471, "Ints"=w472, "Horizontal Binning"=w453, "Vertical Binning"=w454, 5:"in"=w465, 6:"in"=w467, "PSF"=w473, "Pos_Z_Sca"=w452, "ImageArrayLength"=w442, "CCD_Y-X"=w451, "Pos_X_Mir"=w463, "Exposure"=w441, "Pos_Y-Mir"=w464, "Pos_X_Sca"=w470) -> ("error out"=w466:errorcluster)  [unwired: 12 in]
        }
      }
    }
    frame "Area", Default {
      n210 = case shown="\"Mirror\"" w579 {
        selector: w579 -> [w596 w602]
        tunnel: [ctlSeqFNs_PI_SysNr."E710" ("DeviceNr.") ctlSeqFNs_PI_SysNr."E517" ("DeviceNr.")] -> w592
        tunnel: w593 -> [w598 w604]
        tunnel: [w598 w604] -> w583
        tunnel: [w597 w603] -> w591
        tunnel: [w596 w602] -> w590
        tunnel: w582 -> [w595 _]
        tunnel: w581 -> [_ w601]
        tunnel: [w595 w601] -> w580
        tunnel: [w594 w600] -> w577
        tunnel: w576 -> [w594 w600]
        frame "Scanner", Default {
          n211 = global read "GlobalSetConfigurationPhysikalInstruments.vi" "Conn. Axes scanner"() -> (w597:string[])
        }
        frame "Mirror" {
          n212 = global read "GlobalSetConfigurationPhysikalInstruments.vi" "Conn. Axes mirrro"() -> (w603:string[])
        }
      }
      n213 = global read "ModulationNiveaus.vi" "ModulationNiveaus"() -> (w574:dbl[])
      n214 = Array Size(array=w574) -> (size(s)=w573:i32)
      n215 = global read "ccdChipPixels.vi" "CCD Chip Size"() -> (w589:i32)
      n216 = global read "GlobalSetGetTriggerForPointMeasurement.vi" "Frequency"() -> (w585:dbl)
      n217 = global read "SavPath.vi" "SavePath"() -> (w586:path)
      n218 = global read "GlobalSetGetConfigureCamera.vi" "Hbin"() -> (w587:i32)
      n219 = global read "GlobalSetGetConfigureCamera.vi" "Vbin"() -> (w588:i32)
      n220 = case shown="No Error" w583 {
        selector: w583 -> [w652 w1126]
        tunnel: [w642 w1126] -> w575
        tunnel: w591 -> [w667 _]
        tunnel: w590 -> [w665 _]
        tunnel: w592 -> [w666 _]
        tunnel: 0 ("camerahandler") -> [_ _]
        tunnel: w589 -> [_ _]
        tunnel: w588 -> [_ _]
        tunnel: w587 -> [_ _]
        tunnel: w586 -> [_ _]
        tunnel: w585 -> [_ _]
        tunnel: w580 -> [w651 _]
        tunnel: w578 -> [w649 _]
        tunnel: w577 -> [w615 _]
        tunnel: w574 -> [w618 _]
        tunnel: w573 -> [w616 _]
        frame No Error {
          w678 = TRUE ("All axes?")
          w690 = 1000000.0 ("y")
          n221 = global read "IlluminationPatterns.vi" "Illumination Patterns"() -> (w624:T1)
          n222 = case shown="\"Constant Illumination\"" w624 {
            tunnel: w665 -> [w824 w863]
            tunnel: [w823 w862] -> w614
            tunnel: [w822 w861] -> w653
            tunnel: w652 -> [w821 w860]
            tunnel: tag "/Dev3/PFI28" ("destination terminal") -> [w820 w859]
            tunnel: tag "/Dev3/PFI16" ("source terminal") -> [w819 w858]
            tunnel: tag "/Dev3/PFI10" ("source terminal") -> [w818 w857]
            tunnel: tag "/Dev3/PFI32" ("destination terminal") -> [w817 _]
            tunnel: tag "/Dev3/PFI2" ("destination terminal") -> [w816 _]
            tunnel: tag "/Dev3/PFI12" ("destination terminal") -> [w815 _]
            frame "Non Linear Illumniation", Default {
              n223 = case shown="\"Scanner\", Default" w824 {
                selector: w824 -> [w840 w856]
                tunnel: [w840 w856] -> w823
                tunnel: w821 -> [w838 w853]
                tunnel: [w828 w844] -> w822
                tunnel: w818 -> [w836 w854]
                tunnel: w820 -> [w835 w851]
                tunnel: w819 -> [w837 w852]
                tunnel: w817 -> [w827 w843]
                tunnel: w816 -> [w826 w842]
                tunnel: w815 -> [w825 w841]
                frame "Scanner", Default {
                  w832 = 0 items=["no", "yes"] ("invert polarity")
                  w839 = 0 items=["no", "yes"] ("invert polarity")
                  n224 = call <vilib>:"DAQmx Disconnect Terminals.vi"("source terminal"=w836, "destination terminal"=w835, "error in"=w838) -> ("error out"=w834:errorcluster)  [unwired: 12 in]
                  n225 = call <vilib>:"Clear Errors.vi"("error in (no error)"=w834) -> ("error out"=w833:errorcluster)  [unwired: 6 in]
                  n226 = call <vilib>:"DAQmx Connect Terminals.vi"("source terminal"=w837, "destination terminal"=w835, "invert polarity"=w839, "error in"=w833) -> ("error out"=w829:errorcluster)  [unwired: 11 in]
                  n227 = call <vilib>:"DAQmx Disconnect Terminals.vi"("source terminal"=w825, "destination terminal"=w827, "error in"=w829) -> ("error out"=w831:errorcluster)  [unwired: 12 in]
                  n228 = call <vilib>:"Clear Errors.vi"("error in (no error)"=w831) -> ("error out"=w830:errorcluster)  [unwired: 6 in]
                  n229 = call <vilib>:"DAQmx Connect Terminals.vi"("source terminal"=w826, "destination terminal"=w827, "invert polarity"=w832, "error in"=w830) -> ("error out"=w828:errorcluster)  [unwired: 11 in]
                }
                frame "Mirror" {
                  w848 = 0 items=["no", "yes"] ("invert polarity")
                  w855 = 0 items=["no", "yes"] ("invert polarity")
                  n230 = call <vilib>:"DAQmx Disconnect Terminals.vi"("source terminal"=w852, "destination terminal"=w851, "error in"=w853) -> ("error out"=w850:errorcluster)  [unwired: 12 in]
                  n231 = call <vilib>:"Clear Errors.vi"("error in (no error)"=w850) -> ("error out"=w849:errorcluster)  [unwired: 6 in]
                  n232 = call <vilib>:"DAQmx Connect Terminals.vi"("source terminal"=w854, "destination terminal"=w851, "invert polarity"=w855, "error in"=w849) -> ("error out"=w845:errorcluster)  [unwired: 11 in]
                  n233 = call <vilib>:"DAQmx Disconnect Terminals.vi"("source terminal"=w842, "destination terminal"=w843, "error in"=w845) -> ("error out"=w847:errorcluster)  [unwired: 12 in]
                  n234 = call <vilib>:"Clear Errors.vi"("error in (no error)"=w847) -> ("error out"=w846:errorcluster)  [unwired: 6 in]
                  n235 = call <vilib>:"DAQmx Connect Terminals.vi"("source terminal"=w841, "destination terminal"=w843, "invert polarity"=w848, "error in"=w846) -> ("error out"=w844:errorcluster)  [unwired: 11 in]
                }
              }
            }
            frame "Constant Illumination" {
              n236 = case shown="\"Mirror\"" w863 {
                selector: w863 -> [w872 w880]
                tunnel: [w872 w880] -> w862
                tunnel: w860 -> [w869 w878]
                tunnel: [w871 w881] -> w861
                tunnel: w857 -> [w867 w873]
                tunnel: w859 -> [w866 w876]
                tunnel: w858 -> [w868 w877]
                frame "Scanner", Default {
                  w870 = 0 items=["no", "yes"] ("invert polarity")
                  n237 = call <vilib>:"DAQmx Disconnect Terminals.vi"("source terminal"=w867, "destination terminal"=w866, "error in"=w869) -> ("error out"=w865:errorcluster)  [unwired: 12 in]
                  n238 = call <vilib>:"Clear Errors.vi"("error in (no error)"=w865) -> ("error out"=w864:errorcluster)  [unwired: 6 in]
                  n239 = call <vilib>:"DAQmx Connect Terminals.vi"("source terminal"=w868, "destination terminal"=w866, "invert polarity"=w870, "error in"=w864) -> ("error out"=w871:errorcluster)  [unwired: 11 in]
                }
                frame "Mirror" {
                  w879 = 0 items=["no", "yes"] ("invert polarity")
                  n240 = call <vilib>:"DAQmx Disconnect Terminals.vi"("source terminal"=w877, "destination terminal"=w876, "error in"=w878) -> ("error out"=w875:errorcluster)  [unwired: 12 in]
                  n241 = call <vilib>:"Clear Errors.vi"("error in (no error)"=w875) -> ("error out"=w874:errorcluster)  [unwired: 6 in]
                  n242 = call <vilib>:"DAQmx Connect Terminals.vi"("source terminal"=w873, "destination terminal"=w876, "invert polarity"=w879, "error in"=w874) -> ("error out"=w881:errorcluster)  [unwired: 11 in]
                }
              }
            }
          }
          n243 = global read "GlobalSetGetPixelOfRoi.vi" "Stack length"() -> (w691:dbl)
          n244 = global read "GlobalSetGetPixelOfRoi.vi" "Pixel SizeZ"() -> (w658:dbl)
          n245 = global read "GlobalSetGetPixelOfRoi.vi" "Pixel SizeX"() -> (w656:dbl)
          n246 = global read "GlobalSetGetPixelOfRoi.vi" "Pixel SizeY"() -> (w693:dbl)
          n247 = global read "GlobalSetGetPixelOfRoi.vi" "Stack Start"() -> (w692:dbl)
          n248 = global read "GlobalSetGetPixelOfRoi.vi" "Y length"() -> (w688:dbl)
          n249 = global read "GlobalSetGetPixelOfRoi.vi" "X length"() -> (w681:dbl)
          n250 = global read "GlobalSetGetPixelOfRoi.vi" "X Start"() -> (w695:dbl)
          n251 = global read "GlobalSetGetPixelOfRoi.vi" "Y Start"() -> (w694:dbl)
          n252 = global read "ScanDirection.vi" "ScanDirection"() -> (w661:enum32{"X-Y", "X-Z", "Y-Z", "Focus"})
          n253 = Divide(x=w691, y=w658) -> (x/y=w607:dbl)
          n254 = Multiply(x=w695, y=w690) -> (x*y=w613:dbl)
          n255 = Divide(x=w681, y=w656) -> (x/y=w689:dbl)
          n256 = Multiply(x=w658, y=w690) -> (x*y=w685:dbl)
          n257 = Multiply(x=w694, y=w690) -> (x*y=w682:dbl)
          n258 = Multiply(x=w656, y=w690) -> (x*y=w698:dbl)
          n259 = Multiply(x=w692, y=w690) -> (x*y=w699:dbl)
          n260 = Divide(x=w688, y=w693) -> (x/y=w697:dbl)
          n261 = Multiply(x=w693, y=w690) -> (x*y=w700:dbl)
          n262 = case shown="\"Mirror\"" w614 {
            tunnel: w700 -> [w986 w1104]
            tunnel: w607 -> [w985 w1090]
            tunnel: w699 -> [w984 w1103]
            tunnel: w698 -> [w983 w1083]
            tunnel: w613 -> [w982 w1082]
            tunnel: w697 -> [w981 w1088]
            tunnel: [w980 "X-Y"] -> w696
            tunnel: w656 -> [w979 _]
            tunnel: w693 -> [w978 w1086]
            tunnel: w691 -> [w977 _]
            tunnel: [w976 w1101] -> w611
            tunnel: w690 -> [w975 w1100]
            tunnel: w689 -> [w974 w1089]
            tunnel: w688 -> [w973 w1093]
            tunnel: [w972 "1"] -> w655
            tunnel: [w971 w1098] -> w687
            tunnel: [w970 w1097] -> w686
            tunnel: w685 -> [w969 w1096]
            tunnel: w682 -> [w968 w1095]
            tunnel: w681 -> [w967 w1094]
            tunnel: [w966 w1094] -> w680
            tunnel: [w965 w1093] -> w679
            tunnel: [w964 w1092] -> w669
            tunnel: [w963 w1091] -> w668
            tunnel: w653 -> [w962 w1091]
            tunnel: [w961 w1090] -> w664
            tunnel: [w953 w1089] -> w625
            tunnel: [w960 w1088] -> w660
            tunnel: w661 -> [w959 _]
            tunnel: [w958 w1083] -> w659
            tunnel: w658 -> [w957 _]
            tunnel: [w956 w1086] -> w657
            tunnel: [w955 "2"] -> w654
            tunnel: [w954 w1085] -> w650
            tunnel: [_ w1082] -> w612
            frame "Scanner", Default {
              n263 = case shown="\"Focus\"" w959 {
                tunnel: ["1" "2" "3" "1"] -> w972
                tunnel: w962 -> [w1009 w1033 w1056 w1079]
                tunnel: [w1009 w1033 w1056 w1079] -> w963
                tunnel: w981 -> [w996 w1022 _ w1067]
                tunnel: w968 -> [w993 w1012 w1047 w1058]
                tunnel: w986 -> [w1001 w1014 w1049 _]
                tunnel: [w996 w1020 w1042 w1068] -> w960
                tunnel: w985 -> [w995 w1020 w1041 w1068]
                tunnel: w969 -> [w1002 w1024 w1052 w1070]
                tunnel: w984 -> [w994 w1011 w1046 w1059]
                tunnel: w983 -> [w987 w1025 w1053 w1061]
                tunnel: w974 -> [w1003 w1021 _ w1074]
                tunnel: w982 -> [w997 w1013 w1048 w1060]
                tunnel: w979 -> [w991 _ w1039 w1065]
                tunnel: w967 -> [w1004 _ w1043 w1075]
                tunnel: w973 -> [w1007 w1028 _ _]
                tunnel: w978 -> [w992 w1019 _ w1071]
                tunnel: ["X-Y" "Y-Z" "Y-Z" "X-Z"] -> w980
                tunnel: [w1007 w1031 w1043 w1078] -> w965
                tunnel: w977 -> [_ w1031 w1045 w1078]
                tunnel: [w1004 w1028 w1045 w1075] -> w966
                tunnel: [w1006 w1029 w1044 w1077] -> w976
                tunnel: w975 -> [w1005 w1030 w1054 w1076]
                tunnel: [w1003 w1022 w1041 w1074] -> w953
                tunnel: [w995 w1021 w1042 w1067] -> w961
                tunnel: [w1000 w1027 w1035 w1073] -> w971
                tunnel: [w999 w1026 w1038 w1072] -> w970
                tunnel: [w998 w1023 w1051 w1069] -> w964
                tunnel: [w992 w1017 w1039 w1066] -> w958
                tunnel: w957 -> [_ w1017 w1040 w1066]
                tunnel: [w991 w1019 w1040 w1065] -> w956
                tunnel: ["2" "3" "1" "3"] -> w955
                tunnel: [w989 w1016 w1037 w1063] -> w954
                frame "X-Y", Default {
                  w988 = 0.0 ("element")
                  n264 = Multiply(x=w1004, y=w1005) -> (x*y=w1006:dbl)
                  n265 = Build Array(w997, w993, w994) -> (w998:dbl[])
                  n266 = Build Array(w988, w988, w1002) -> (w999:dbl[])
                  n267 = Build Array(w987, w988, w988) -> (w989:dbl[])
                  n268 = Build Array(w988, w1001, w988) -> (w1000:dbl[])
                }
                frame "Y-Z" {
                  w1015 = 0.0 ("element")
                  n269 = Multiply(x=w1028, y=w1030) -> (x*y=w1029:dbl)
                  n270 = Build Array(w1013, w1012, w1011) -> (w1023:dbl[])
                  n271 = Build Array(w1015, w1015, w1024) -> (w1027:dbl[])
                  n272 = Build Array(w1025, w1015, w1015) -> (w1026:dbl[])
                  n273 = Build Array(w1015, w1014, w1015) -> (w1016:dbl[])
                }
                frame "Focus" {
                  w1042 = 1.0
                  w1036 = 0.0 ("element")
                  n274 = Multiply(x=w1045, y=w1054) -> (x*y=w1044:dbl)
                  n275 = Build Array(w1048, w1047, w1046) -> (w1051:dbl[])
                  n276 = Build Array(w1036, w1036, w1052) -> (w1035:dbl[])
                  n277 = Build Array(w1053, w1036, w1036) -> (w1037:dbl[])
                  n278 = Build Array(w1036, w1049, w1036) -> (w1038:dbl[])
                }
                frame "X-Z" {
                  w1062 = 0.0 ("element")
                  n279 = Multiply(x=w1075, y=w1076) -> (x*y=w1077:dbl)
                  n280 = Build Array(w1060, w1058, w1059) -> (w1069:dbl[])
                  n281 = Build Array(w1062, w1062, w1070) -> (w1073:dbl[])
                  n282 = Build Array(w1061, w1062, w1062) -> (w1063:dbl[])
                  n283 = Build Array(w1062, w1071, w1062) -> (w1072:dbl[])
                }
              }
            }
            frame "Mirror" {
              w1084 = 0.0 ("element")
              n284 = Multiply(x=w1094, y=w1100) -> (x*y=w1101:dbl)
              n285 = Build Array(w1082, w1095, w1103) -> (w1092:dbl[])
              n286 = Build Array(w1084, w1084, w1096) -> (w1097:dbl[])
              n287 = Build Array(w1083, w1084, w1084) -> (w1085:dbl[])
              n288 = Build Array(w1084, w1104, w1084) -> (w1098:dbl[])
            }
          }
          n289 = call "TMN?.vi"("System no."=w666, "Axes to query"=w667, "All axes?"=w678, "Axis identifier?"=w678, "error in"=w668) -> ("Minimum travel limit"=w675:dbl[], "error out"=w677:errorcluster)  [unwired: 13 in]
          n290 = call "TMX?.vi"("System no."=w666, "Axes to query"=w667, "All axes?"=w678, "Axis identifier?"=w678, "error in"=w677) -> ("Maximum travel limit"=w674:dbl[], "error out"=w676:errorcluster)  [unwired: 13 in]
          n291 = In Range and Coerce(upper limit=w674, x=w669, lower limit=w675) -> (coerced(x)=w671:dbl[], In Range?=w673:bool[])
          n292 = case shown="\"Mirror\"" w614 {
            tunnel: w673 -> [w948 w949]
            tunnel: [w945 w952] -> w672
            frame "Scanner", Default {
              n293 = Index Array(array=w948) -> (element #1=w947:bool, element #2=w946:bool, element #3=w944:bool)  [unwired: 3 in]
              n294 = Compound Arithmetic op=AND(w947, w946, w944) -> (w945:bool)
            }
            frame "Mirror" {
              n295 = Index Array(array=w949) -> (element #1=w951:bool, element #2=w950:bool)  [unwired: 2 in]
              n296 = And(x=w951, y=w950) -> (x .and. y?=w952:bool)
            }
          }
          n297 = case shown="True" w672 {
            tunnel: w671 -> [_ w1108]
            tunnel: w676 -> [w1105 w1118]
            tunnel: [w1106 w1116] -> w670
            tunnel: w667 -> [_ w1110]
            tunnel: w666 -> [_ w1115]
            tunnel: w651 -> [_ w1112]
            tunnel: w614 -> [_ w1111]
            frame False {
              n298 = call "Display Message to User"("error in (no error)"=w1105) -> ("error out"=w1106:errorcluster)  [unwired: 9 in, 1 out]
            }
            frame True {
              n299 = case shown="\"Mirror\"" w1111 {
                tunnel: [w1120 string[] ["1", "2"] ("Conn. Axes mirrro")] -> w1109
                tunnel: w1110 -> [w1120 _]
                tunnel: w1108 -> [w1119 w1123]
                tunnel: [w1119 w1121] -> w1107
                frame "Scanner", Default {
                }
                frame "Mirror" {
                  n300 = Index Array(array=w1123) -> (element #1=w1124:dbl, element #2=w1122:dbl)  [unwired: 2 in]
                  n301 = Build Array(w1124, w1122) -> (w1121:dbl[])
                }
              }
              n302 = call "MOV.vi"("System no."=w1115, "Axes to move"=w1109, "Position values"=w1107, "No.of digits"=w1112, "error in"=w1118) -> ("error out"=w1117:errorcluster)  [unwired: 14 in]
              n303 = call "General wait for movement to stop.vi"("System no."=w1115, "Axes to wait for"=w1109, "All axes?"=FALSE, "Additional wait time, ms"=u32 1000, "error in"=w1117) -> ("error out"=w1116:errorcluster)  [unwired: 13 in, 1 out]
            }
          }
          n304 = call "POS?.vi"("System no."=w666, "Axes to query"=w667, "error in"=w670) -> ("Position"=w610:dbl[], "error out"=w684:errorcluster)  [unwired: 15 in]
          n305 = case shown="\"Mirror\"" w614 {
            tunnel: w684 -> [w920 w943]
            tunnel: [w919 w942] -> w683
            tunnel: w610 -> [w917 w936]
            tunnel: w661 -> [w918 _]
            tunnel: [w917 w937] -> w609
            tunnel: [_ w936] -> w608
            frame "Scanner", Default {
              n306 = Index Array(array=w917) -> (element #1=w922:dbl, element #2=w921:dbl, element #3=w923:dbl)  [unwired: 3 in]
              n307 = case shown="\"X-Y\", Default" w918 {
                tunnel: [w927 w931 w935] -> w919
                tunnel: w920 -> [w927 w931 w935]
                tunnel: w921 -> [w925 w928 w932]
                tunnel: w922 -> [w926 w930 w933]
                tunnel: w923 -> [w924 w929 w934]
                frame "X-Y", Default {
                  n308 = global write "GlobalSetGetPositionParameters.vi" "ind POS X 2"(w926) -> ()
                  n309 = global write "GlobalSetGetPositionParameters.vi" "ind POS  Y 2"(w925) -> ()
                  n310 = global write "GlobalSetGetPositionParameters.vi" "ind POS Z 2"(w924) -> ()
                }
                frame "Y-Z" {
                  n311 = global write "GlobalSetGetPositionParameters.vi" "ind POS X 2"(w930) -> ()
                  n312 = global write "GlobalSetGetPositionParameters.vi" "ind POS  Y 2"(w928) -> ()
                  n313 = global write "GlobalSetGetPositionParameters.vi" "ind POS Z 2"(w929) -> ()
                }
                frame "X-Z" {
                  n314 = global write "GlobalSetGetPositionParameters.vi" "ind POS X 2"(w933) -> ()
                  n315 = global write "GlobalSetGetPositionParameters.vi" "ind POS  Y 2"(w932) -> ()
                  n316 = global write "GlobalSetGetPositionParameters.vi" "ind POS Z 2"(w934) -> ()
                }
              }
            }
            frame "Mirror" {
              n317 = Index Array(array=w936) -> (element #1=w939:dbl, element #2=w938:dbl)  [unwired: 2 in]
              n318 = global write "GlobalSetGetPositionParameters.vi" "ind POS X rad 2"(w939) -> ()
              n319 = global write "GlobalSetGetPositionParameters.vi" "ind POS  Y rad 2"(w938) -> ()
              n320 = global read "GlobalSetConfigurationPhysikalInstruments.vi" "Conn. Axes scanner"() -> (w940:string[])
              n321 = call "POS?.vi"("System no."=ctlSeqFNs_PI_SysNr."E710" ("DeviceNr."), "Axes to query"=w940, "error in"=w943) -> ("Position"=w937:dbl[], "error out"=w942:errorcluster)  [unwired: 15 in]
            }
          }
          n322 = case shown="\"Stepwise\"" w649 {
            selector: w649 -> [w884 w915]
            tunnel: w611 -> [w896 _]
            tunnel: [w895 w916] -> w645
            tunnel: w683 -> [w894 w916]
            tunnel: w625 -> [w893 _]
            tunnel: [w892 _] -> w663
            tunnel: [w891 _] -> w662
            tunnel: w614 -> [w890 _]
            tunnel: w660 -> [w889 _]
            tunnel: w659 -> [w888 _]
            tunnel: w657 -> [w887 _]
            tunnel: w655 -> [w886 _]
            tunnel: w654 -> [w885 _]
            tunnel: [w884 w915] -> w620
            tunnel: w615 -> [w883 _]
            tunnel: w612 -> [w882 _]
            frame "Linear", Default {
              n323 = case shown="\"Mirror\"" w890 {
                tunnel: [w905 w914] -> w895
                tunnel: w896 -> [w904 w913]
                tunnel: [w903 w912] -> w891
                tunnel: w893 -> [_ _]
                tunnel: w889 -> [w899 w908]
                tunnel: w894 -> [w902 w911]
                tunnel: w886 -> [w901 w910]
                tunnel: [w900 w909] -> w892
                tunnel: w888 -> [_ _]
                tunnel: w887 -> [w897 w906]
                tunnel: w885 -> [_ _]
                tunnel: w883 -> [w898 w907]
                tunnel: w882 -> [_ _]
                frame "Scanner", Default {
                  n324 = call "E710_InitialisationOfWaveScan.vi"("amplitude"=w904, "Fast Axis"=w901, "Slow Axis Steps"=w899, "error in"=w902, "FastAxisStepsize"=w897, "kineticexposure"=w898) -> ("scan time for 1 line/sec"=w903:dbl, "scan time for 1 area/sec 2"=w900:dbl, "error out 2"=w905:errorcluster)  [unwired: 7 in]
                }
                frame "Mirror" {
                  n325 = call "E517_InitialisatOfWaveScan.vi"("amplitude"=w913, "Fast Axis"=w910, "Slow Axis Steps"=w908, "error in"=w911, "FastAxisStepsize"=w906, "kineticexposure"=w907) -> ("scan time for 1 line/sec"=w912:dbl, "scan time for 1 area/sec 2"=w909:dbl, "error out 2"=w914:errorcluster)  [unwired: 7 in]
                }
              }
            }
            frame "Stepwise" {
            }
          }
          n326 = global read "AOTF_NonLinearLinesOnOff.vi" "LineOnOff"() -> (w619:bool[])
          n327 = global write "MesaurementTime.vi" "Mesaurement line"(w662) -> ()
          n328 = global write "MesaurementTime.vi" "Mesaurement time area"(w663) -> ()
          n329 = case shown="\"Stepwise\"" w620 {
            tunnel: w645 -> [w764 w793]
            tunnel: [w763 w792] -> w644
            tunnel: w619 -> [w762 _]
            tunnel: [w761 _] -> w641
            tunnel: [w760 _] -> w640
            tunnel: [w759 _] -> w639
            tunnel: [w758 _] -> w638
            tunnel: [w757 _] -> w637
            tunnel: [w756 _] -> w636
            tunnel: [w755 _] -> w635
            tunnel: [w754 _] -> w634
            tunnel: [w753 _] -> w633
            tunnel: [w752 _] -> w632
            tunnel: [w751 _] -> w631
            tunnel: [w750 _] -> w630
            tunnel: [w749 _] -> w629
            tunnel: [w748 _] -> w628
            tunnel: [w747 _] -> w627
            tunnel: [w746 _] -> w626
            tunnel: w625 -> [w745 w788]
            tunnel: w618 -> [w744 w789]
            tunnel: w624 -> [w743 _]
            tunnel: [_ w794] -> w617
            tunnel: [w742 _] -> w606
            frame "Linear", Default {
              n330 = case shown="\"Non Linear Illumniation\", Default" w743 {
                tunnel: w764 -> [w786 w787]
                tunnel: [w785 w787] -> w763
                tunnel: w762 -> [w784 _]
                tunnel: [w783 _] -> w761
                tunnel: [w782 _] -> w760
                tunnel: [w781 _] -> w759
                tunnel: [w780 _] -> w758
                tunnel: [w779 _] -> w757
                tunnel: [w778 _] -> w756
                tunnel: [w777 _] -> w755
                tunnel: [w776 _] -> w754
                tunnel: [w766 _] -> w753
                tunnel: [w775 _] -> w752
                tunnel: [w774 _] -> w751
                tunnel: [w773 _] -> w750
                tunnel: [w772 _] -> w749
                tunnel: [w771 _] -> w748
                tunnel: [w770 _] -> w747
                tunnel: [w769 _] -> w746
                tunnel: w745 -> [w768 _]
                tunnel: w744 -> [w767 _]
                tunnel: [w765 _] -> w742
                frame "Non Linear Illumniation", Default {
                  n331 = call "AOTF_NonLinCreateTasks.vi"("LineOnOff"=w784, "AmplitudenNiveaus"=w767, "error in (no error)"=w786, "FastAxisSteps"=w768) -> ("405out"=w765:refnum<k21>, "task 8"=w775:refnum<k21>, "task 4"=w771:refnum<k21>, "LineOnOff[5]"=w778:bool, "task 2"=w769:refnum<k21>, "LineOnOff[4]"=w779:bool, "task 3"=w770:refnum<k21>, "LineOnOff[3]"=w780:bool, "task 6"=w773:refnum<k21>, "LineOnOff[2]"=w781:bool, "task1"=w766:refnum<k21>, "LineOnOff[7]"=w776:bool, "task5"=w772:refnum<k21>, "LineOnOff[6]"=w777:bool, "task 7"=w774:refnum<k21>, "LineOnOff[0]"=w783:bool, "LineOnOff[1]"=w782:bool, "error out"=w785:errorcluster)  [unwired: 6 in]
                }
                frame "Constant Illumination" {
                }
              }
            }
            frame "Stepwise" {
              n332 = Index Array(array=w789, index=0) -> (element=w790:dbl)
              n333 = for {
                tunnel: [w803] -> w794 mode=indexing
                tunnel: w788 -> [w802]
                tunnel: w790 -> [w798]
                shift-right: [w797] -> w792
                shift-left: w793 -> [w796]
                tunnel: w789 -> [w795] mode=indexing
                n334 = Divide(x=w795, y=w798) -> (x/y=w801:dbl)
                n335 = Multiply(x=10000.0, y=w802) -> (x*y=w799:dbl)
                n336 = for {
                  N: w799 -> [_]
                  shift-right: [w811] -> w797
                  shift-left: w796 -> [w811]
                  tunnel: w801 -> [w806]
                  tunnel: w798 -> [w810]
                  tunnel: [w809] -> w803 mode=indexing
                  tunnel: w795 -> [w804]
                  i -> [w812]
                  n337 = Increment(x=w812) -> (x+1=w807:i32)
                  n338 = Quotient & Remainder(x=w807, y=w806) -> (x-y*floor(x/y)=w805:dbl)  [unwired: 1 out]
                  n339 = Equal To 0?(x=w805) -> (x = 0?=w808:bool)
                  n340 = case shown="True" w808 {
                    tunnel: w810 -> [w813 _]
                    tunnel: [w813 w814] -> w809
                    tunnel: w804 -> [_ w814]
                    frame False {
                    }
                    frame True {
                    }
                  }
                }
              }
            }
          }
          n341 = call "RunMeasurement.vi"("NumberOfDigits"=w651, "DeviceNr."=w666, "Image Fast Axis"=w680, "Image Slow Axis"=w679, "Number Fast Axis Steps"=w625, "Number of Stackslides"=w664, "ScanOrientation"=w696, "error in"=w644, "StartPointScanner"=w609, "Fast Axis"=w655, "Fast axis delta"=w650, "Slow Axis"=w654, "Number Slow Axis  Steps"=w660, "Slow Axis Delta"=w687, "Stack Axis Delta"=w686, "kinetic"=w615, "LineOnOff"=w619, "scan time for 1 line/sec"=w662, "Modulation#"=w616, "ArrayOfWaves"=w617, "StartPositionMirror"=w608) -> ("error out"=w643:errorcluster)  [unwired: 6 in]
          n342 = case shown="\"Linear\", Default" w620 {
            tunnel: w643 -> [w720 w741]
            tunnel: [w719 w741] -> w642
            tunnel: w641 -> [w718 _]
            tunnel: w640 -> [w717 _]
            tunnel: w639 -> [w716 _]
            tunnel: w638 -> [w715 _]
            tunnel: w637 -> [w714 _]
            tunnel: w636 -> [w713 _]
            tunnel: w635 -> [w712 _]
            tunnel: w634 -> [w711 _]
            tunnel: w633 -> [w710 _]
            tunnel: w632 -> [w709 _]
            tunnel: w631 -> [w708 _]
            tunnel: w630 -> [w707 _]
            tunnel: w629 -> [w706 _]
            tunnel: w628 -> [w705 _]
            tunnel: w627 -> [w704 _]
            tunnel: w626 -> [w703 _]
            tunnel: w624 -> [w702 _]
            tunnel: w606 -> [w701 _]
            frame "Linear", Default {
              n343 = case shown="\"Non Linear Illumniation\", Default" w702 {
                tunnel: w720 -> [w739 w740]
                tunnel: [w738 w740] -> w719
                tunnel: w718 -> [w737 _]
                tunnel: w717 -> [w736 _]
                tunnel: w716 -> [w735 _]
                tunnel: w715 -> [w734 _]
                tunnel: w714 -> [w733 _]
                tunnel: w713 -> [w732 _]
                tunnel: w712 -> [w731 _]
                tunnel: w711 -> [w730 _]
                tunnel: w710 -> [w729 _]
                tunnel: w709 -> [w728 _]
                tunnel: w708 -> [w727 _]
                tunnel: w707 -> [w726 _]
                tunnel: w706 -> [w725 _]
                tunnel: w705 -> [w724 _]
                tunnel: w704 -> [w723 _]
                tunnel: w703 -> [w722 _]
                tunnel: w701 -> [w721 _]
                frame "Non Linear Illumniation", Default {
                  n344 = call "AOTF_NonLinKillTasks.vi"("Refnum in"=w729, "task out"=w722, "LineOnOff[3]"=w734, "task out 3"=w724, "LineOnOff[4]"=w733, "task out 7"=w728, "task out 4"=w725, "error in (no error)"=w739, "LineOnOff[2]"=w735, "task out 6"=w727, "task out 2"=w723, "LineOnOff[0]"=w737, "LineOnOff[1]"=w736, "LineOnOff[5]"=w732, "task out 5"=w726, "405Pico"=w721, "LineOnOff[6]"=w731, "LineOnOff[7]"=w730) -> ("error out"=w738:errorcluster)  [unwired: 9 in]
                }
                frame "Constant Illumination" {
                }
              }
            }
            frame "Stepwise" {
            }
          }
        }
        frame Error {
        }
      }
    }
  }
  n345 = global read "IlluminationPatterns.vi" "Illumination Patterns"() -> (w8:T1)
  n346 = case shown="\"Constant Illumination\"" w8 {
    tunnel: w11 -> [w1128 w1133]
    tunnel: [w1127 w1133] -> w10
    frame "Non Linear Illumniation", Default {
      n347 = Concatenate Strings("daughter enable" ("string"), "\r") -> (w1131:string)
      n348 = call "CTI_AOTF.vi"("error in"=w1128, "String"=w1131, "VISA resource name 2"=refnum<visa-resource-name> "USB0::0x16C7::0x0001::NI-VISA-20001::RAW") -> ("error out"=w1127:errorcluster)  [unwired: 7 in, 1 out]
    }
    frame "Constant Illumination" {
    }
  }
  "error out" <- w10
